vi "ini_sesion.vi"(8 "error in (no error)":errorcluster, 11 "5785_2_x_200MHz in":refnum<class "5785_2_x_200MHz.lvclass">) -> (0 "error out":errorcluster, 3 "5785_2_x_200MHz out":refnum<class "5785_2_x_200MHz.lvclass">)   [LabVIEW 2021, in "5785_2_x_200MHz.lvclass"]
uses:
  5785_2_x_200MHz.lvclass
  5785_2_x_200MHz.lvclass/5785_2_x_200MHz.ctl
  <instrlib>/FlexRIO/API/Host/v1/NI FlexRIO/API/Reference Clock Source.ctl
  <instrlib>/FlexRIO/API/Host/v1/NI FlexRIO API v1.lvlib
  <resource>/objmgr/niflexrioapiStream.rc
  <resource>/objmgr/niflexrioapi.rc
  <vilib>/rvi/interface/nirviOpenFPGA/nirviOpenFPGA.xnode
  FPGA Bitfiles/ChaimPersonality_pulse_X_2_11.lvbitx
  <vilib>/rvi/interface/nirviMethod/nirviMethod.xnode
  <vilib>/FPGAPlugInAG/Dynamic/niLvFpga_ConfigureFifo_Dynamic.vi
  <vilib>/rvi/errors/niLvFpgaMergeErrorWithErrorCode.vi
  <resource>/objmgr/niflexrioapiChannel.rc
  <vilib>/rvi/interface/nirviReadWriteControl/nirviReadWriteControl.xnode
  NiFpgaLv.dll
  <vilib>/Utility/error.llb/Error Cluster From Error Code.vi
  <vilib>/rvi/interface/Simulation/niFpgaSimulationCallBeginRW.vi
  <vilib>/rvi/errors/niLvFpgaAdjustHostInterfaceError.vi
  <vilib>/FPGAPlugInAG/Dynamic/niLvFpga_StopFifo_Dynamic.vi
  <instrlib>/FlexRIO/API/Host/v1/NI FlexRIO/API/Configure Reference Clock.vi
  <instrlib>/FlexRIO/API/Host/v1/NI FlexRIO/API/Get Property Reference - Fpga Small.vi
  <vilib>/FPGAPlugInAG/PXIe-5785 (KU060)/niLvFpga_Open_PXIe-5785 (KU060).vi
  <vilib>/rvi/interface/common/dynamic/niFpgaDynamicAddResources.vi
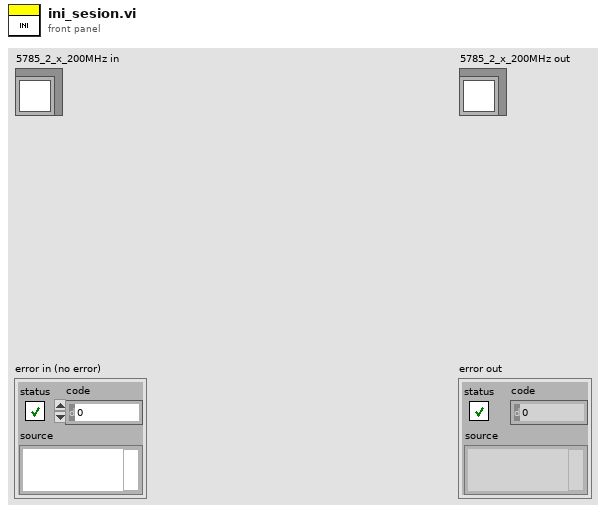
[diagram p1: front panel]
types:
  T1 = typedef "nirio_resource_hc.ctl" = tag
  T2 = typedef "NI FlexRIO API v1.lvlib/Reference Clock Source.ctl" = i32
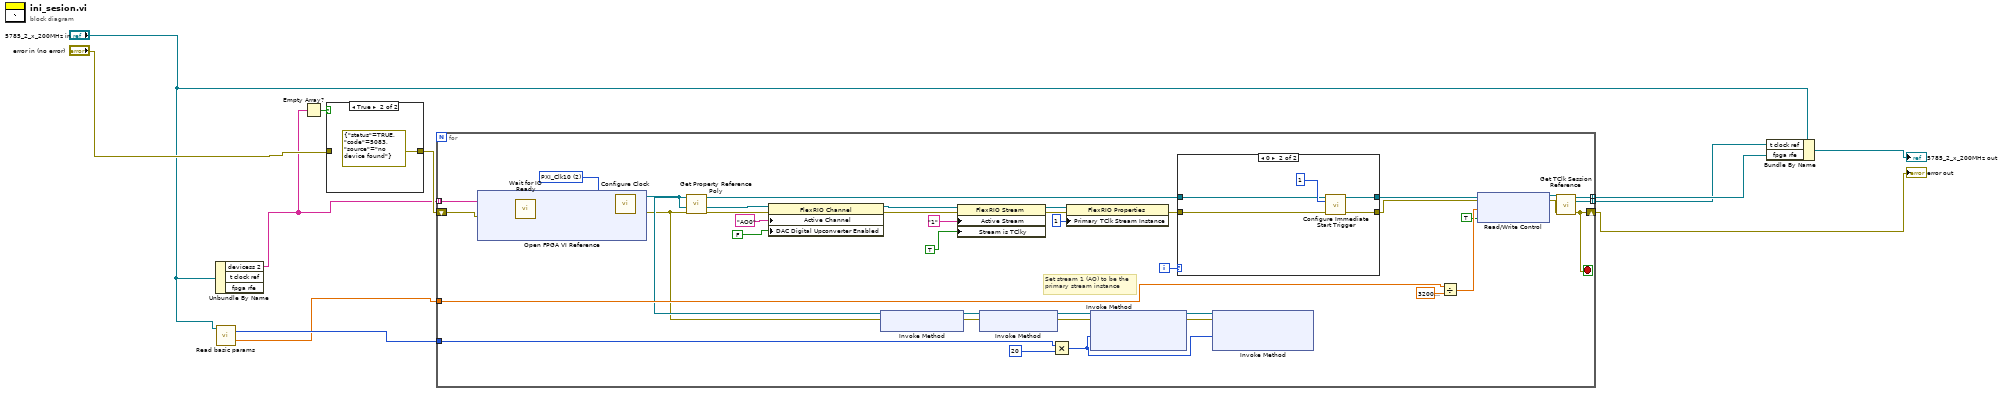
[diagram p0: block diagram]
diagram:
  n1 = Unbundle By Name("5785_2_x_200MHz in") -> ("devicess 2"=w3:T1[])  [unwired: 2 out]
  n2 = call-dynamic "Read basic params.vi"("device_type in"="5785_2_x_200MHz in") -> ("buffer size"=w5:u32, "center frequency (Hz)"=w4:dbl)  [unwired: 13 in, 4 out]
  n3 = Empty Array?(array=w3) -> (empty?=w9:bool)
  n4 = case shown="True" w9 {
    tunnel: [w12 errorcluster {"status"=TRUE, "code"=5083, "source"="no device found"} ("error in (no error)")] -> w8
    tunnel: "error in (no error)" -> [w12 _]
    frame False {
    }
    frame True {
    }
  }
  n5 = for {
    tunnel: [w50] -> w11 mode=indexing
    shift-right: [w29] -> w1
    shift-left: w8 -> [w44]
    tunnel: [w49] -> w10 mode=indexing
    tunnel: w3 -> [w33] mode=indexing
    tunnel: w4 -> [w21]
    tunnel: w5 -> [w14]
    i -> [w47]
    stop <- w29 stop-if-true
    w32 = T2 2 items=["Default", "Onboard", "PXI_Clk10", "External", "None", "Baseboard Reference"] ("reference clock source")
    # "Set stream 1 (AO) to be the\nprimary stream instance"
    n6 = xnode "Open FPGA VI Reference"("error in"=w44, "resource name"=w33) -> ("FPGA VI Reference Out"=w46:refnum<k20>, "error out"=w45:errorcluster)
    n7 = call <instrlib>:"Wait for IO Ready.vi"("fpga interface in"=w46, "error in"=w45) -> ("fpga interface out"=w31:refnum<k20>, "error out"=w30:errorcluster)  [unwired: 10 in, 2 out]
    n8 = call-poly <instrlib>:"Configure Clock.vi"("fpga interface in"=w31, "reference clock source"=w32, "error in"=w30) -> ("fpga interface out"=w20:refnum<k20>, "error out"=w19:errorcluster)  [unwired: 11 in]
    n9 = call-poly <instrlib>:"Get Property Reference Poly.vi"("error in (no error)"=w19, "fpga interface in"=w20) -> ("error out"=w36:errorcluster, "property reference"=w37:refnum<k20>)  [unwired: 4 in, 1 out]
    n10 = property class="FlexRIO Channel"(reference=w37, error in=w36, "Active Channel"="AO0", "DAC Digital Upconverter Enabled"=FALSE ("Analog Output:DAC Digital Upconverter Enabled")) -> (reference out=w35:refnum<k20>, error out=w34:errorcluster)
    n11 = xnode "Invoke Method"("FPGA VI Reference In"=w20, "error in"=w19) -> ("FPGA VI Reference Out"=w17:refnum<k20>, "error out"=w18:errorcluster)
    n12 = property class="FlexRIO Stream"(reference=w35, error in=w34, "Active Stream"="1", "Stream is TClky"=TRUE ("Configuration:Stream is TClky")) -> (reference out=w53:refnum<k20>, error out=w52:errorcluster)
    n13 = xnode "Invoke Method"("FPGA VI Reference In"=w17, "error in"=w18) -> ("FPGA VI Reference Out"=w15:refnum<k20>, "error out"=w16:errorcluster)
    n14 = Multiply(x=w14, y=u32 20) -> (x*y=w41:u32)
    n15 = property class="FlexRIO Properties"(reference=w53, error in=w52, "Primary TClk Stream Instance"=1 ("Device:Primary TClk Stream Instance")) -> (error out=w48:errorcluster)  [unwired: 1 out]
    n16 = xnode "Invoke Method"("FPGA VI Reference In"=w15, "error in"=w16, "Requested Depth"=w41) -> ("FPGA VI Reference Out"=w43:refnum<k20>, "error out"=w42:errorcluster)  [unwired: 1 out]
    n17 = case shown="0" w47 {
      tunnel: w20 -> [w57 w61]
      tunnel: [w57 w60] -> w28
      tunnel: [w56 w59] -> w25
      tunnel: w48 -> [w56 w58]
      frame 1, Default {
      }
      frame 0 {
        n18 = call <instrlib>:"Configure Immediate Start Trigger.vi"("fpga interface in"=w61, "trigger instance"=u32 1, "error in"=w58) -> ("fpga interface out"=w60:refnum<k20>, "error out"=w59:errorcluster)  [unwired: 10 in, 1 out]
      }
    }
    n19 = xnode "Invoke Method"("FPGA VI Reference In"=w43, "error in"=w42, "Requested Depth"=w41) -> ()  [unwired: 3 out]
    n20 = Divide(x=w21, y=3200000000.0) -> (x/y=w23:dbl)
    n21 = xnode "Read/Write Control"("FPGA VI Reference In"=w28, "error in"=w25, "frequency shift 1"=w23, "reset system clock"=TRUE) -> ("FPGA VI Reference Out"=w27:refnum<k20>, "error out"=w26:errorcluster)
    n22 = call <instrlib>:"Get TClk Session Reference.vi"("fpga interface in"=w27, "error in"=w26) -> ("fpga interface out"=w50:refnum<k20>, "tclk session reference"=w49:refnum<k20>, "error out"=w29:errorcluster)  [unwired: 11 in]
  }
  "error out" <- w1
  n23 = Bundle By Name(cluster="5785_2_x_200MHz in", "t clock ref"=w10, "fpga rfe"=w11) -> (→"5785_2_x_200MHz out":refnum<class "5785_2_x_200MHz.lvclass">)
